vi "Replace Array Subset.vi"   [LabVIEW 2016, in "JSON Value.lvclass"]
doc: "Replaces an element or subarray in an array at the point you specify in index."
uses:
  JSON Value.lvclass
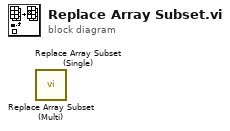
[diagram p0: block diagram]
diagram:
  n1 = call "Replace Array Subset (Multi).vi"() -> ()  [unwired: 15 in, 1 out]
  n2 = call "Replace Array Subset (Single).vi"() -> ()  [unwired: 14 in, 2 out]
